vi "Plattform_Move_CT.vi"(10 "vr , vl":i32[](array[numeric])) -> (2 "Command":string)   [LabVIEW 2017]
uses:
  sobot structures/SoBot_CommandTypes.ctl
  sobot structures/Plattform_Command.ctl
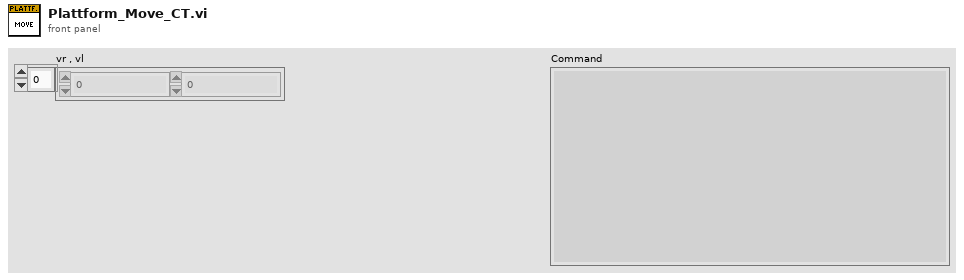
[diagram p1: front panel]
types:
  T1 = typedef "Plattform_Command.ctl" = enum16{"Plattform_Move", "Plattform_GetDrivingData", "Plattform_GetLivetimeData"}
  T2 = typedef "SoBot_CommandTypes.ctl" = enum16{"General_Command", "XY_Command", "Z_Command", "Plattform_Command"}
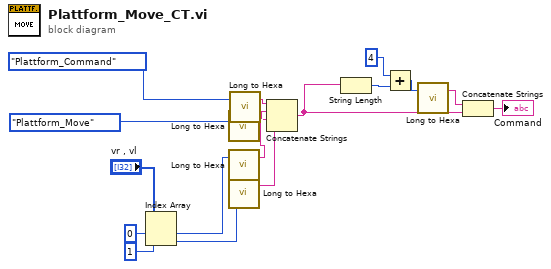
[diagram p0: block diagram]
diagram:
  n1 = Index Array(array="vr , vl", index #1=0 ("index"), index #2=1 ("index")) -> (element #1=w5:i32, element #2=w4:i32)
  n2 = call "Long to Hexa.vi"("Long"=Plattform_Command."Plattform_Move" ("Plattform_Command")) -> ("Hexa"=w16:string)  [unwired: 2 in]
  n3 = call "Long to Hexa.vi"("Long"=w5) -> ("Hexa"=w8:string)  [unwired: 2 in]
  n4 = call "Long to Hexa.vi"("Long"=w4) -> ("Hexa"=w7:string)  [unwired: 2 in]
  n5 = call "Long to Hexa.vi"("Long"=SoBot_CommandTypes."Plattform_Command" ("SoBot_CommandTypes")) -> ("Hexa"=w17:string)  [unwired: 2 in]
  n6 = Concatenate Strings(w17, w16, w8, w7) -> (w11:string)
  n7 = String Length(string=w11) -> (length=w15:i32)
  n8 = Add(x=4, y=w15) -> (x+y=w13:i32)
  n9 = call "Long to Hexa.vi"("Long"=w13) -> ("Hexa"=w12:string)  [unwired: 2 in]
  n10 = Concatenate Strings(w12, w11) -> (→"Command":string)
